vi "labels.set.vi"(8 "error in (no error)":errorcluster, 10 "labels":set{string}(c389), 11 "labels in":refnum<class "labels.lvclass">) -> (0 "error out":errorcluster, 3 "labels out":refnum<class "labels.lvclass">)   [LabVIEW 2020, in "nominal types.lvlib" / "labels.lvclass"]
uses:
  labels.lvclass
  labels.lvclass/labels.ctl
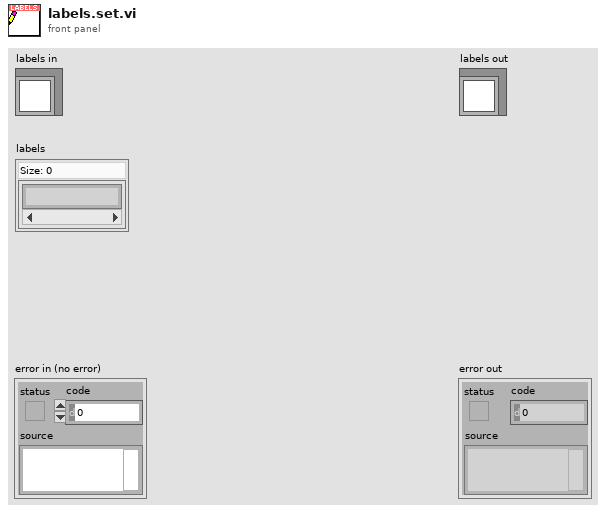
[diagram p1: front panel]
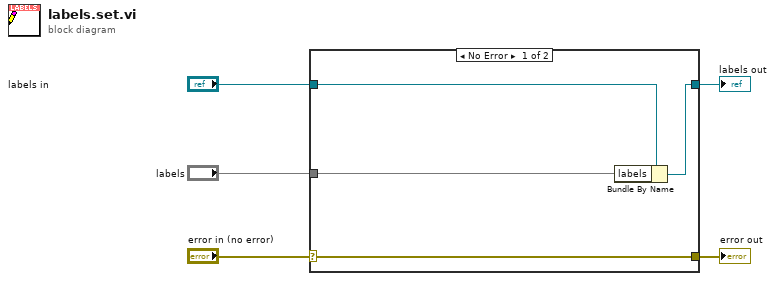
[diagram p0: block diagram]
diagram:
  n1 = case shown="No Error" "error in (no error)" {
    selector: "error in (no error)" -> [w9 w10]
    tunnel: [w9 w10] -> w4
    tunnel: [w7 w11] -> w2
    tunnel: "labels in" -> [w8 w11]
    tunnel: "labels" -> [w6 _]
    frame No Error {
      n2 = Bundle By Name(cluster=w8, "labels"=w6) -> (w7:refnum<class "labels.lvclass">)
    }
    frame Error {
    }
  }
  "error out" <- w4
  "labels out" <- w2
